vi "MALT24VI Output Set Several.vi"(8 "error in":errorcluster, 9 "State":bool, 10 "State Map":u8[](array[numeric]) format="%02x", 11 "Address":i32) -> (0 "error out":errorcluster)   [LabVIEW 2018, in "AltonTech MALT200817.lvlib"]
uses:
  <instrlib>/AltonTech MALT/AltonTech MALT200817.lvlib
  <instrlib>/AltonTech MALT/Public/Types/MALT CardTypes.ctl
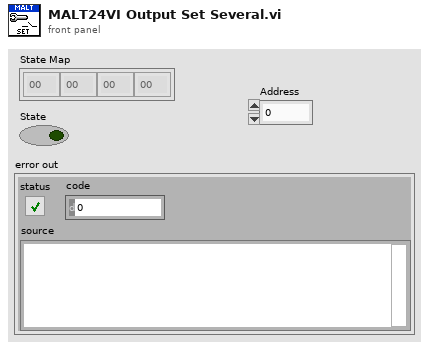
[diagram p1: front panel]
types:
  T1 = typedef "AltonTech MALT200817.lvlib/MALT CardTypes.ctl" = enum32{"-", "YAV90832", "YAV904X8", "MALT132", "YAV91616", "YAV90PIN", "YAV90096", "YAV90HVT", "YAV90CLR", "YAV90128", "YAV90PNE", "YAVCANCON", "YAV91775", "YAV90XXX", "YAV90MMU", "H730050", "H710060", "H710061", "YAV90304", "MMI", "YAV90060", "MALT160T", "YAV90059", "Not Defined"}
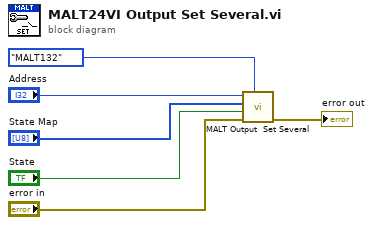
[diagram p0: block diagram]
diagram:
  n1 = call <instrlib>:"MALT Output  Set Several.vi"("MALT CardType"=MALT_CardTypes."MALT132", "error in"="error in", "State"="State", "State Map"="State Map", "Address"="Address") -> ("error out"=→"error out":errorcluster)  [unwired: 6 in]
